vi "Update comments exp.vi"(8 "error in (no error)":errorcluster, 10 "Commentaires":string, 11 "Control-Client in":refnum<class "Control-Client.lvclass">) -> (0 "error out":errorcluster, 3 "Control-Client out":refnum<class "Control-Client.lvclass">)   [LabVIEW 2019, in "Control-Client.lvclass"]
uses:
  Control-Client.lvclass
  Experiments/Experiment.lvclass
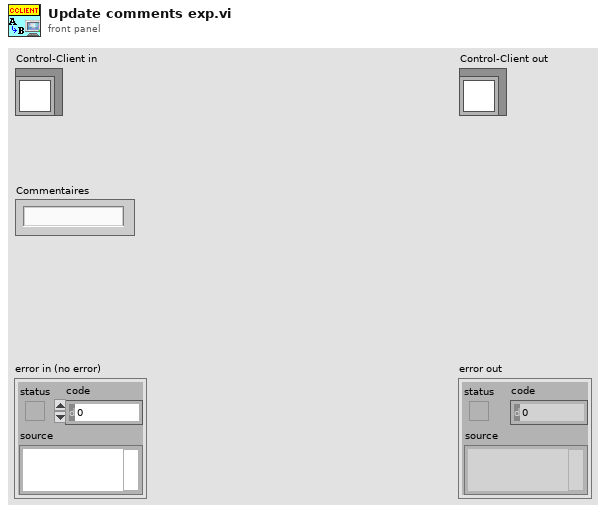
[diagram p1: front panel]
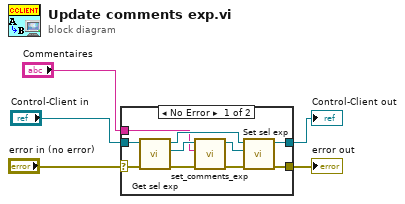
[diagram p0: block diagram]
diagram:
  n1 = case shown="No Error" "error in (no error)" {
    selector: "error in (no error)" -> [w9 w17]
    tunnel: [w6 w17] -> w4
    tunnel: [w12 w16] -> w2
    tunnel: "Control-Client in" -> [w13 w16]
    tunnel: "Commentaires" -> [w8 _]
    frame No Error {
      n2 = call "Get sel exp.vi"("error in (no error)"=w9, "Control-Client in"=w13) -> ("error out"=w10:errorcluster, "Sel experiment"=w15:refnum<class "Experiment.lvclass">, "Control-Client out"=w11:refnum<class "Control-Client.lvclass">)  [unwired: 7 in]
      n3 = call "set_comments_exp.vi"("error in (no error)"=w10, "Comments"=w8, "Experiment.lvclass in"=w15) -> ("error out"=w14:errorcluster, "Experiment.lvclass out"=w7:refnum<class "Experiment.lvclass">)  [unwired: 7 in]
      n4 = call "Set sel exp.vi"("error in (no error)"=w14, "Experiment"=w7, "Control-Client in"=w11) -> ("error out"=w6:errorcluster, "Control-Client out"=w12:refnum<class "Control-Client.lvclass">)  [unwired: 7 in]
    }
    frame Error {
    }
  }
  "error out" <- w4
  "Control-Client out" <- w2
